vi "AndorCreaterErrorCluster.vi"() -> (3 "Array":cluster{i32, string}[](array[cluster]))   [LabVIEW 2018, in "AndorOWN.lvlib"]
uses:
  AndorOWN.lvlib
panel:
  in  "String":string="DRV_ERROR_CODES 20001\nDRV_P1INVALID 20066\nDRV_SUCCESS 20002\nDRV_P2INVALID 20067\nDRV_VXDNOTINSTALLED 20003\nDRV_P3INVALID 20068\nDRV_ERROR_SCAN 20004\nDRV_P4INVALID 20069\nDRV_ERROR_CHECK_SUM 20005\nDRV_INIERROR 20070\nDRV_ERROR_FILELOAD 20006\nDRV_COFERROR 20071\nDRV_UNKNOWN_FUNCTION 20007\nDRV_ACQUIRING 20072\nDRV_ERROR_VXD_INIT 20008\nDRV_IDLE 20073\nDRV_ERROR_ADDRESS 20009\nDRV_TEMPCYCLE 20074\nDRV_ERROR_PAGELOCK 20010\nDRV_NOT_INITIALIZED 20075\nDRV_ERROR_PAGE_UNLOCK 20011\nDRV_P5INVALID 20076\nDRV_ERROR_BOARDTEST 20012\nDRV_P6INVALID 20077\nDRV_ERROR_ACK 20013\nDRV_INVALID_MODE 20078\nDRV_ERROR_UP_FIFO 20014\nDRV_INVALID_FILTER 20079\nDRV_ERROR_PATTERN 20015\nDRV_I2CERRORS 20080\nDRV_ACQUISITION_ERRORS 20017\nDRV_DRV_I2CDEVNOTFOUND 20081\nDRV_ACQ_BUFFER 20018\nDRV_I2CTIMEOUT 20082\nDRV_ACQ_DOWNFIFO_FULL 20019\nDRV_P7INVALID 20083\nDRV_PROC_UNKNOWN_INSTRUCTION 20020\nDRV_USBERROR 20089\nDRV_ILLEGAL_OP_CODE 20021\nDRV_IOCERROR 20090\nDRV_KINETIC_TIME_NOT_MET 20022\nDRV_NOT_SUPPORTED 20091\nDRV_KINETIC_TIME_NOT_MET 20022\nDRV_USB_INTERRUPT_ENDPOINT_ERROR 20093\nDRV_ACCUM_TIME_NOT_MET 20023\nDRV_RANDOM_TRACK_ERROR 20094\nDRV_NO_NEW_DATA 20024\nDRV_INVALID_TRIGGER_MODE 20095\nDRV_SPOOLERROR 20026\nDRV_LOAD_FIRMWARE_ERROR 20096\nDRV_TEMPERATURE_CODES 20033\nDRV_DIVIDE_BY_ZERO_ERROR 20097\nDRV_TEMPERATURE_OFF 20034\nDRV_INVALID_RINGEXPOSURES 20098\nDRV_TEMPERATURE_NOT_STABILIZED 20035\nDRV_BINNING_ERROR 20099\nDRV_TEMPERATURE_STABILIZED 20036\nDRV_ERROR_NOCAMERA 20990\nDRV_TEMPERATURE_NOT_REACHED 20037\nDRV_NOT_SUPPORTED 20991\nDRV_TEMPERATURE_OUT_RANGE 20038\nDRV_NOT_AVAILABLE 20992\nDRV_TEMPERATURE_NOT_SUPPORTED 20039 \nDRV_ERROR_MAP 20115\nDRV_TEMPERATURE_DRIFT 20040\nDRV_ERROR_UNMAP 20116\nDRV_GENERAL_ERRORS 20049\nDRV_ERROR_MDL 20117\nDRV_INVALID_AUX 20050\nDRV_ERROR_UNMDL 20118\nDRV_COF_NOTLOADED 20051\nDRV_ERROR_BUFFSIZE 20119\nDRV_FPGAPROG 20052\nDRV_ERROR_NOHANDLE 20121\nDRV_FLEXERROR 20053\nDRV_GATING_NOT_AVAILABLE 20130\nDRV_GPIBERROR 20054\nDRV_FPGA_VOLTAGE_ERROR 20131\nDRV_DATATYPE 20064\nDRV_BINNING_ERROR 20099\nDRV_DRIVER_ERRORS 20065\nDRV_INVALID_AMPLIFIER 20100"
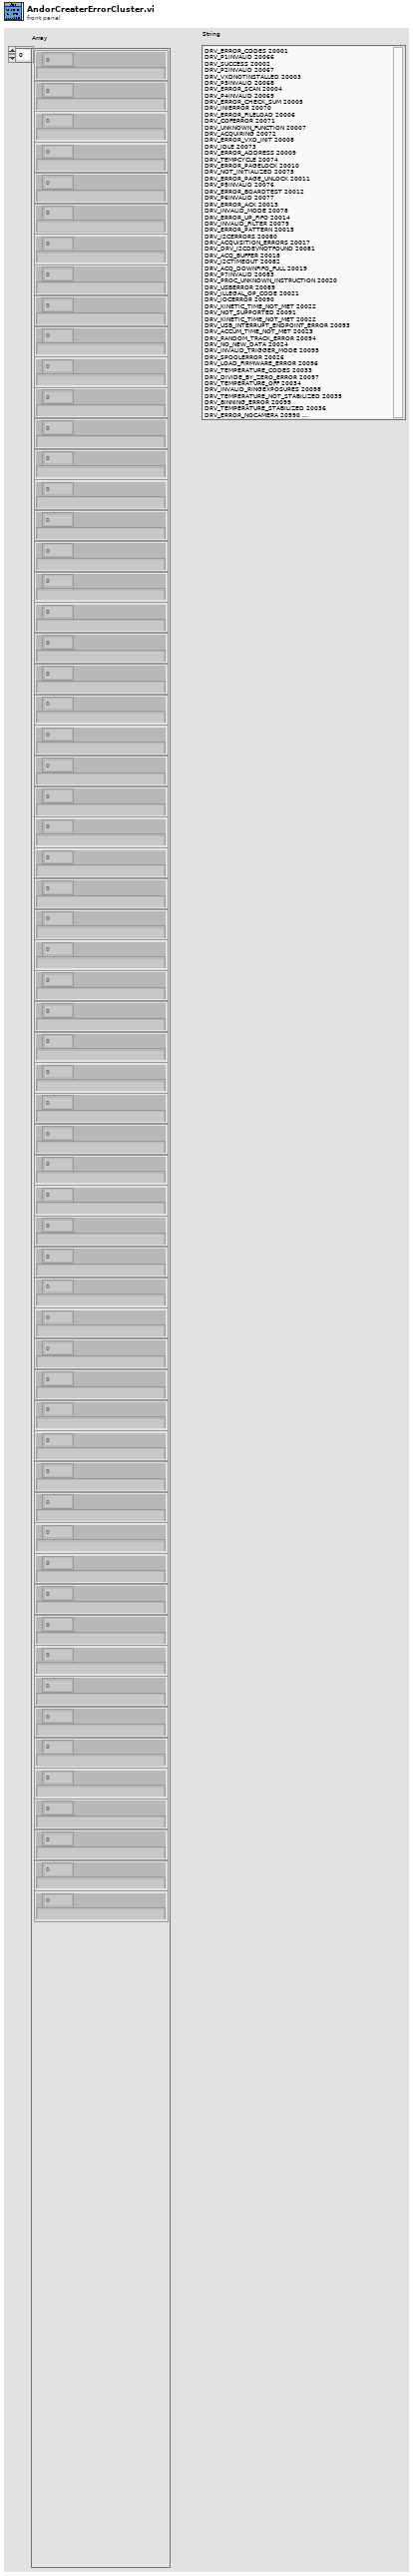
[diagram p1: front panel]
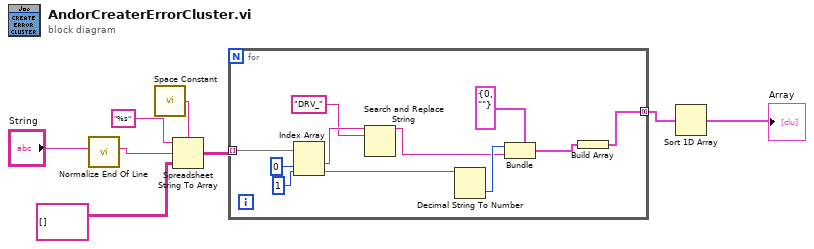
[diagram p0: block diagram]
diagram:
  n1 = call <vilib>:"Normalize End Of Line.vi"("string in"="String") -> ("string out"=w2:string)  [unwired: 7 in]
  n2 = call <vilib>:"Space Constant.vi"() -> ("String"=w7:string)
  n3 = Spreadsheet String To Array(delimiter (Tab)=w7, format string="%s", spreadsheet string=w2, array type (2D Dbl)=string[][] []) -> (array=w4:string[][])
  n4 = for {
    tunnel: w4 -> [w16] mode=indexing
    tunnel: [w17] -> w5 mode=concatenating
    n5 = Index Array(array=w16, index #1=0 ("index"), index #2=1 ("index")) -> (element #1=w10:string, element #2=w12:string)
    n6 = Search and Replace String(input string=w10, search string="DRV_") -> (result string=w11:string)  [unwired: 6 in, 3 out]
    n7 = Decimal String To Number(string=w12) -> (number=w18:i32)  [unwired: 2 in, 1 out]
    n8 = Bundle(cluster=cluster{i32, string} {0, ""}, w18, w11) -> (w19:cluster{i32, string})
    n9 = Build Array(w19) -> (w17:cluster{i32, string}[])
  }
  n10 = Sort 1D Array(array=w5) -> (sorted array=→"Array":cluster{i32, string}[])
